vi "Generate colour map.vi"() -> ()   [LabVIEW 2020]
panel:
  out "Blue":u8[](array[numeric])
  out "Green":u8[](array[numeric])
  out "Red":u8[](array[numeric])
  in  "Number of images":i32
  # "R = 18, G = 255, B = 85"
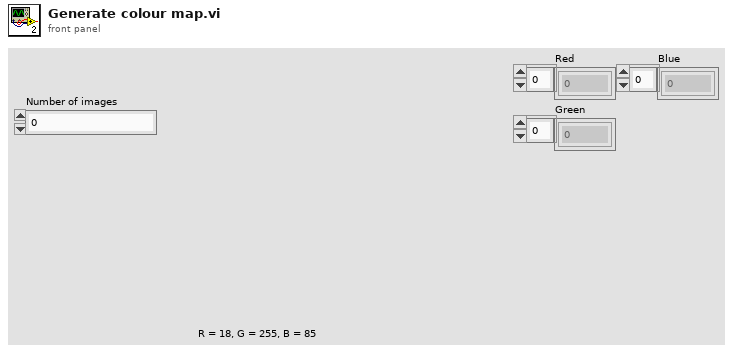
[diagram p1: front panel]
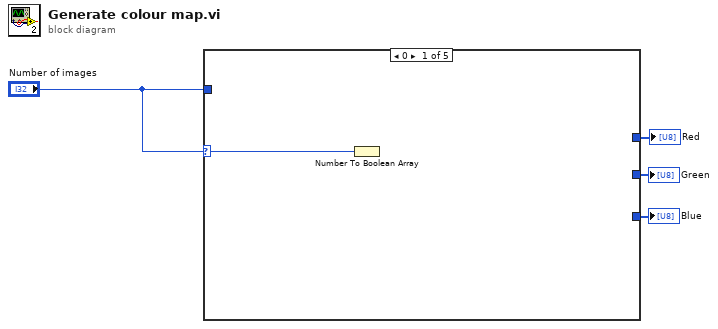
[diagram p0: block diagram]
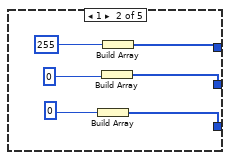
[diagram p2: hidden frame]
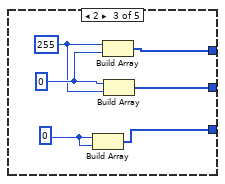
[diagram p3: hidden frame]
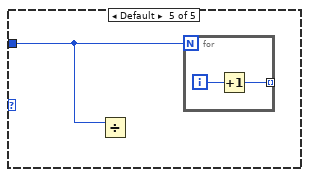
[diagram p5: hidden frame]
diagram:
  n1 = case shown="0" "Number of images" {
    selector: "Number of images" -> [w5 _ _ _ _]
    tunnel: "Number of images" -> [_ _ _ _ w18]
    tunnel: [_ w10 w17 _ _] -> w3
    tunnel: [_ w6 w13 _ _] -> w2
    tunnel: [_ w8 w12 _ _] -> w1
    frame 0 {
      n2 = Number To Boolean Array(number=w5) -> ()  [unwired: 1 out]
    }
    frame 1 {
      n3 = Build Array(u8 0) -> (w8:u8[])
      n4 = Build Array(u8 0) -> (w6:u8[])
      n5 = Build Array(u8 255) -> (w10:u8[])
    }
    frame 2 {
      w16 = u8 0
      w15 = u8 0
      w14 = u8 255
      n6 = Build Array(w16, w16) -> (w12:u8[])
      n7 = Build Array(w14, w15) -> (w17:u8[])
      n8 = Build Array(w15, w14) -> (w13:u8[])
    }
    frame 3 {
    }
    frame Default {
      n9 = Divide(x=w18) -> ()  [unwired: 1 in, 1 out]
      n10 = for {
        N: w18 -> [_]
        tunnel: [w19] -> _ mode=indexing
        i -> [w20]
        n11 = Increment(x=w20) -> (x+1=w19:i32)
      }
    }
  }
  "Red" <- w3
  "Green" <- w2
  "Blue" <- w1
